vi "Set_freq.vi"(8 "error in (no error)":errorcluster, 9 "Div bit rate":dbl=32.0, 10 "Carrier":dbl=13560.0, 11 "RF in":refnum<class "Store.lvclass">) -> (0 "error out":errorcluster, 3 "RF out":refnum<class "Store.lvclass">)   [LabVIEW 2019]
uses:
  Store.lvclass
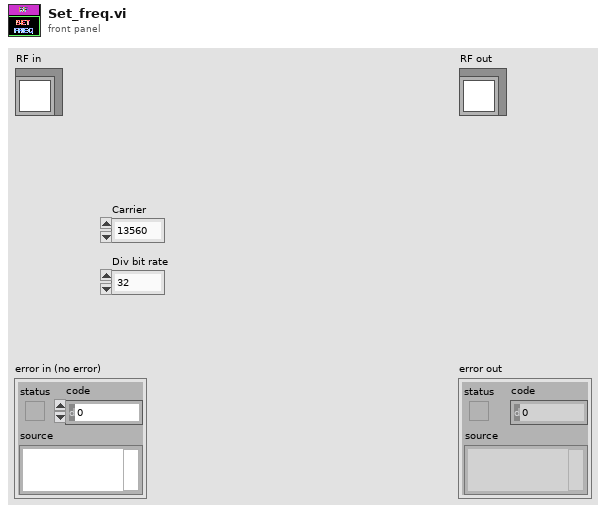
[diagram p1: front panel]
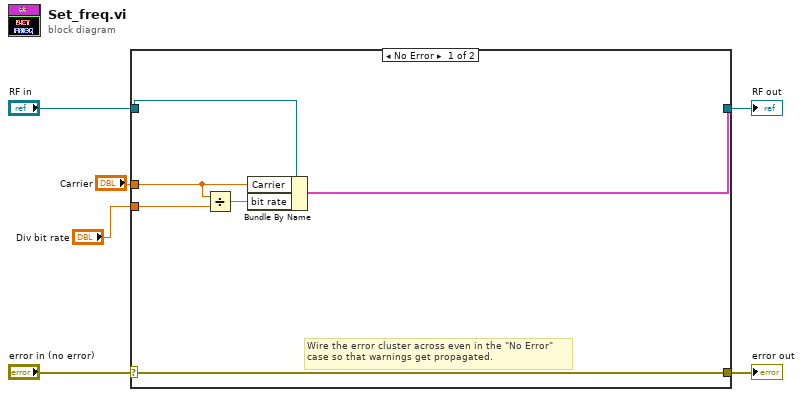
[diagram p0: block diagram]
diagram:
  n1 = case shown="No Error" "error in (no error)" {
    selector: "error in (no error)" -> [w12 w14]
    tunnel: [w12 w14] -> w5
    tunnel: [w8 w13] -> w3
    tunnel: "RF in" -> [w7 w13]
    tunnel: "Carrier" -> [w10 _]
    tunnel: "Div bit rate" -> [w9 _]
    frame No Error {
      # "Wire the error cluster across even in the \"No Error\"\ncase so that warnings get propagated."
      n2 = Divide(x=w10, y=w9) -> (x/y=w11:dbl)
      n3 = Bundle By Name(cluster=w7, "Carrier"=w10, "bit rate"=w11) -> (w8:cluster{})
    }
    frame Error {
    }
  }
  "error out" <- w5
  "RF out" <- w3
